vi "(SubVI)I2C_16Bit-8Bit_Read_Single.vi"(5 "Log Ref":refnum<vi>, 7 "Clock":T1=enum."400kHz", 8 "error in (no error)":errorcluster caption="에러 입력(에러 없음)", 10 "Address":u16, 11 "ID":u8) -> (0 "error out":errorcluster caption="에러 출력", 2 "Log":string, 3 "Read Data":u8)   [LabVIEW 2020]
uses:
  Controls/(Ctrl)I2C_Clock.ctl
  Serial/Controls/(Ctrl)Serial_Write Read Option.ctl
  Controls/(Ctrl)I2C_RW.ctl
  Controls/(Ctrl)I2C_Data Size.ctl
  Variables/(Var)System Variables.vi
  Serial/Instance VIs/(SubVI)Serial_Write-Read.vi
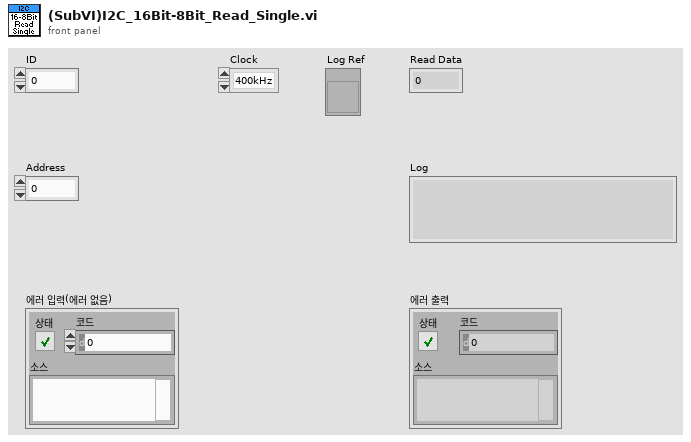
[diagram p1: front panel]
types:
  T1 = typedef "(Ctrl)I2C_Clock.ctl" = enum8{"1MHz", "2MHz", "3MHz", "400kHz"}
  T2 = typedef "(Ctrl)I2C_Data Size.ctl" = enum16{"8Bit_8Bit", "16Bit_16Bit", "16Bit_8Bit"}
  T3 = typedef "(Ctrl)I2C_RW.ctl" = enum16{"Read", "Write"}
  T4 = typedef "(Ctrl)Serial_Write Read Option.ctl" = cluster{"Echo Request":bool, "Header Verification":bool, "Checksum Verification":bool, "User Code Verifiaction":bool}
  T5 = typedef "IC I2C Clock Rate.ctl" = enum8{"50khz", "100khz", "400khz", "1Mhz", "1.2Mhz"}
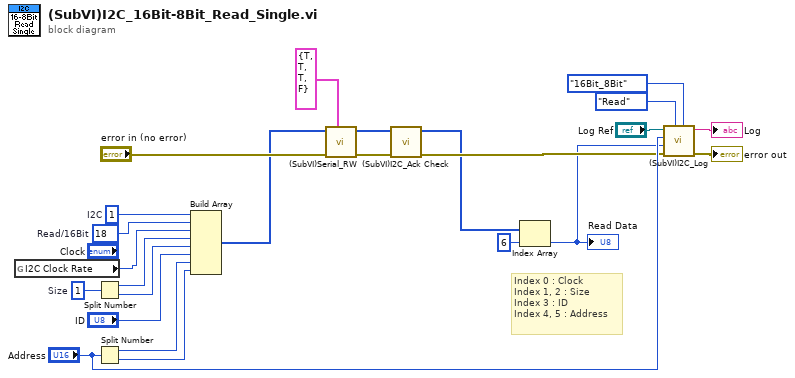
[diagram p0: block diagram]
diagram:
  w15 = u16 1  # Size
  w22 = u8 18  # Read/16Bit
  w23 = u8 1  # I2C
  # "Index 0 : Clock\nIndex 1, 2 : Size\nIndex 3 : ID\nIndex 4, 5 : Address"
  n1 = global read "(Var)System Variables.vi" "I2C Clock Rate"() -> (w1:T5)
  n2 = Split Number(x=w15) -> (hi(x)=w21:u8, lo(x)=w20:u8)
  n3 = Split Number(x="Address") -> (hi(x)=w16:u8, lo(x)=w17:u8)
  n4 = Build Array(w23, w22, w1, w21, w20, "ID", w16, w17) -> (w4:u8[])
  n5 = call-poly "(SubVI)Serial_RW.vi"("Option"=T4 {"Echo Request"=TRUE, "Header Verification"=TRUE, "Checksum Verification"=TRUE, "User Code Verifiaction"=FALSE}, "error in (no error)"="error in (no error)", "Data to Write"=w4) -> ("error out"=w6:errorcluster, "Read Data"=w14:u8[])  [unwired: 6 in, 1 out]
  n6 = call "(SubVI)I2C_Ack Check.vi"("에러 입력(에러 없음)"=w6, "Read Data"=w14) -> ("에러 출력"=w5:errorcluster, "Read Data Out"=w3:u8[])  [unwired: 8 in]
  n7 = Index Array(array=w3, index=6 ("인덱스")) -> (element=w2:u8)
  "Read Data" <- w2
  n8 = call "(SubVI)I2C_Log.vi"("Data Size"=(Ctrl)I2C_Data_Size."16Bit_8Bit", "R/W"=(Ctrl)I2C_RW."Read", "error in (no error)"=w5, "Data"=w2, "Address"="Address", "Log Ref"="Log Ref") -> ("error out"=→"error out":errorcluster, "Log"=→"Log":string)  [unwired: 4 in]
